vi "SanitizePathComponents.vi"(1 "PathComponentsIn":string[](array[string])) -> (0 "SanitizedComponentsOut":string[](array[string]))   [LabVIEW 2022 SP3]
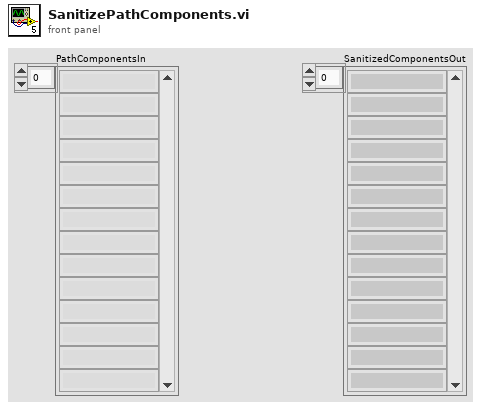
[diagram p1: front panel]
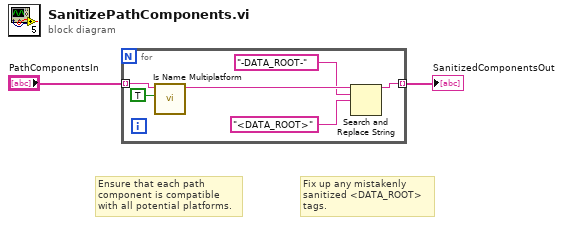
[diagram p0: block diagram]
diagram:
  # "Fix up any mistakenly\nsanitized <DATA_ROOT>\ntags."
  # "Ensure that each path\ncomponent is compatible\nwith all potential platforms."
  n1 = for {
    tunnel: [w5] -> w1 mode=indexing
    tunnel: "PathComponentsIn" -> [w7] mode=indexing
    n2 = call <vilib>:"Is Name Multiplatform.vi"("filename must be valid on all platforms (F)"=TRUE ("name must work for all platforms (F)"), "filename"=w7) -> ("suggested filename"=w6:string)  [unwired: 5 in, 4 out]
    n3 = Search and Replace String(input string=w6, search string="-DATA_ROOT-", replace string="<DATA_ROOT>" ("replace string (\"\")")) -> (result string=w5:string)  [unwired: 5 in, 3 out]
  }
  "SanitizedComponentsOut" <- w1
